vi "Traverse_to_Traverse_Collision.vi"(5 "Current Position  (Tun Coord)":sgl[](array[numeric])=[0.0, 100.0, 40.0], 7 "Traverse Name":string, 10 "Simulate/Run":T1=enum."Run VI", 11 "New Position (Tun Coord)":sgl[](array[numeric])=[0.0, 100.0, 40.0]) -> (1 "Error String":string)   [LabVIEW 2022 SP3]
uses:
  Controls/User_Specific_mode.ctl
  Route mapping/Exclude_cluster.ctl
  Route mapping/Box_size.ctl
  Route mapping/Exclusion_type.ctl
  Globals/Preference_global.vi
panel:
  in  "Max  (Xtunnel - Xtrav1) mm":dbl=2500.0
  out "Z Difference":sgl format="%#.0f"
  out "Xtrav1 - Xtunnel":sgl format="%#.0f"
  out "Static Trav Position (Tun)":sgl[](array[numeric]) format="%#.0f"
  in  "Z Difference":dbl=500.0
  in  "Max  (Xtrav1 - Xtunnel) mm":dbl=30.0
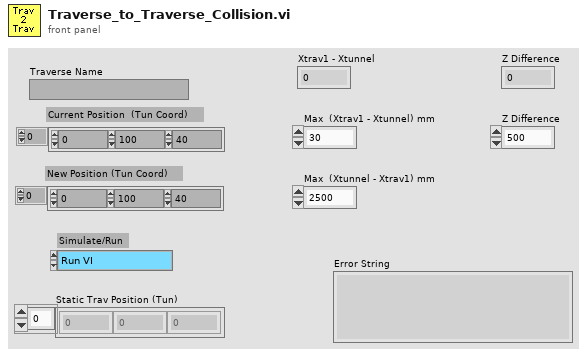
[diagram p1: front panel]
types:
  T1 = typedef "User_Specific_mode.ctl" = enum16{"Check VI only", "Run VI"}
  T2 = typedef "Exclude_cluster.ctl" = cluster{"Sizes":T3, "Name":string, "Exclude Type":T4}
  T3 = typedef "Box_size.ctl" = cluster{"Max":sgl, "Min":sgl}[]
  T4 = typedef "Exclusion_type.ctl" = enum16{"Exclude completely", "Allow only vertical moves"}
  T5 = enum16{"Load setup from excel file", "Save setup to excel file"}
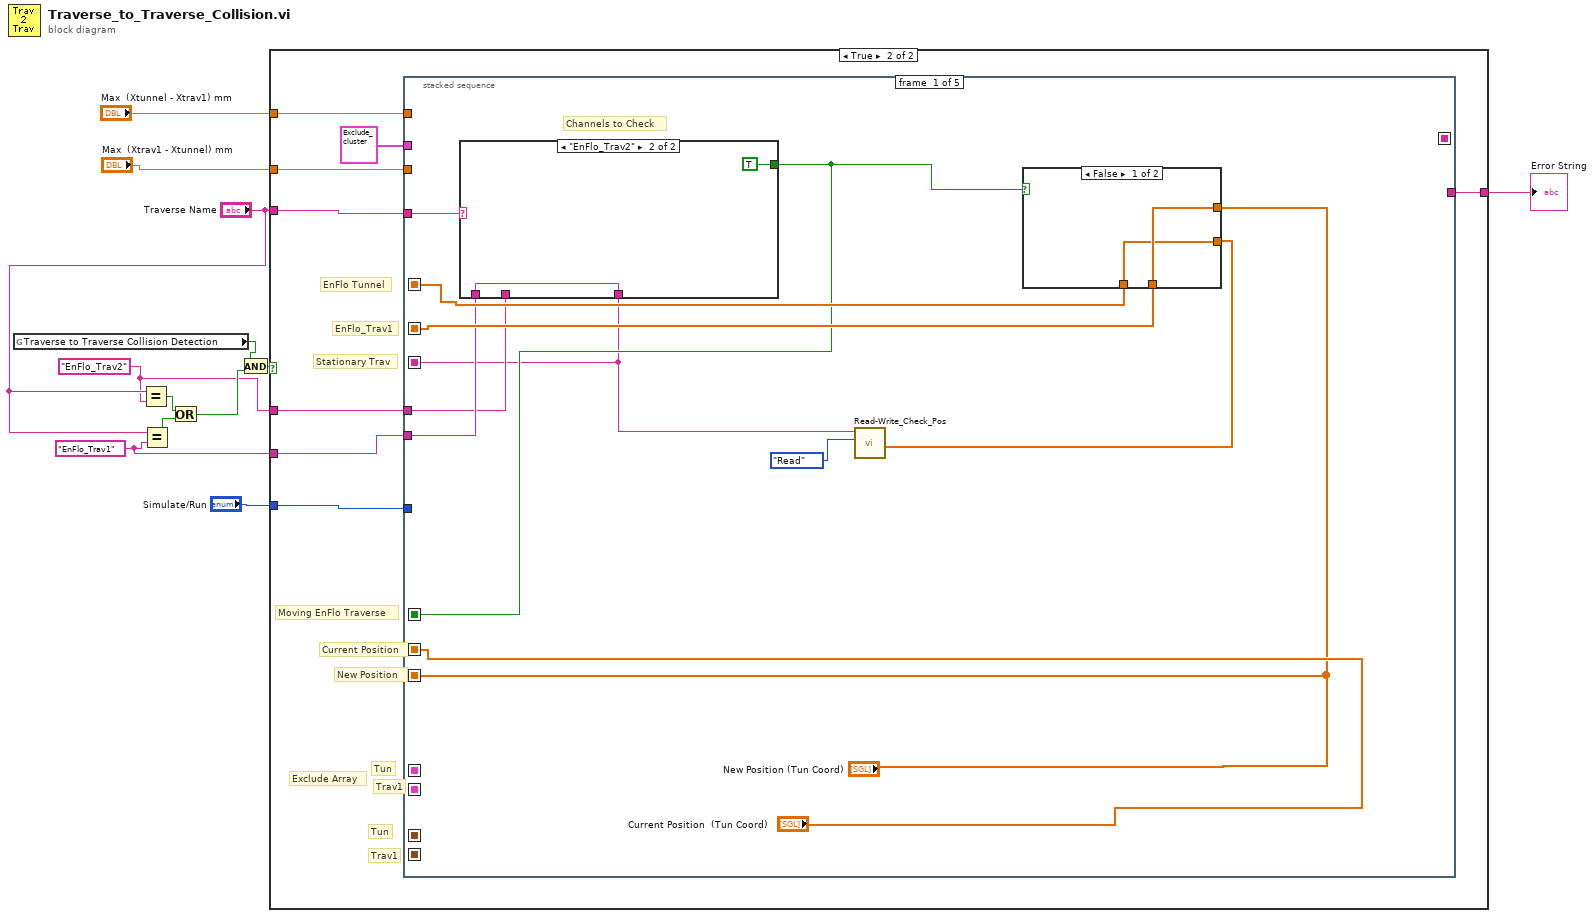
[diagram p0: block diagram]
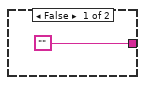
[diagram p2: hidden frame]
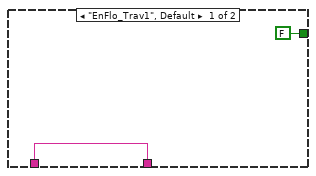
[diagram p4: hidden frame]
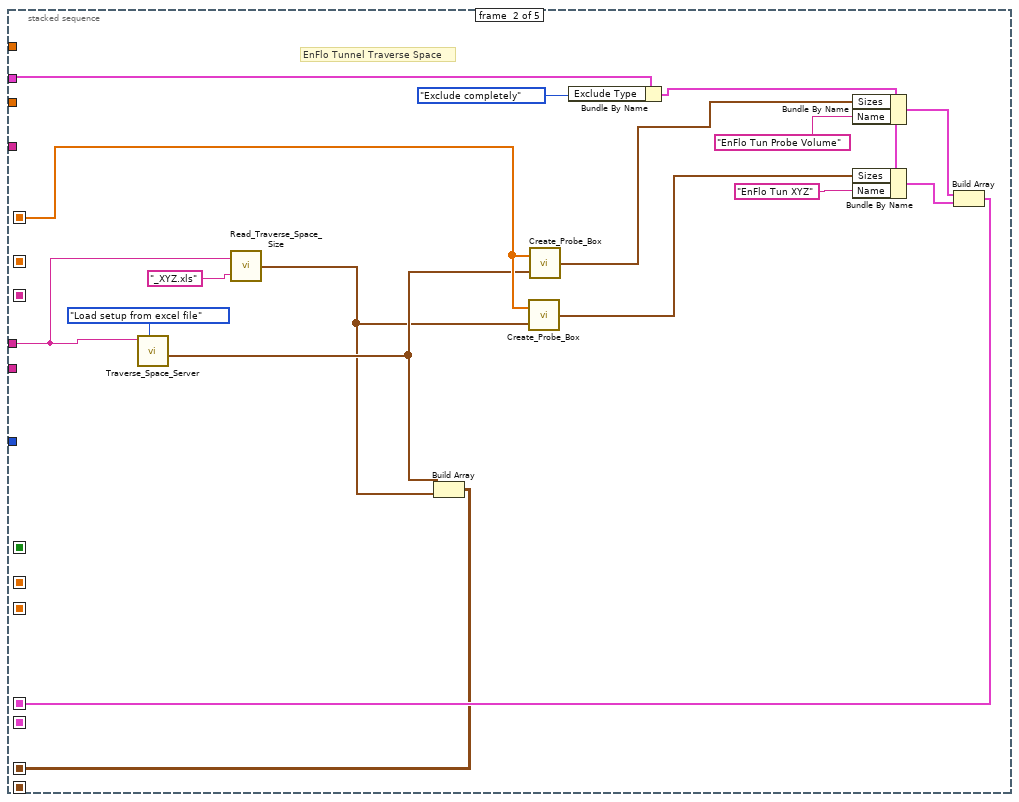
[diagram p5: hidden frame]
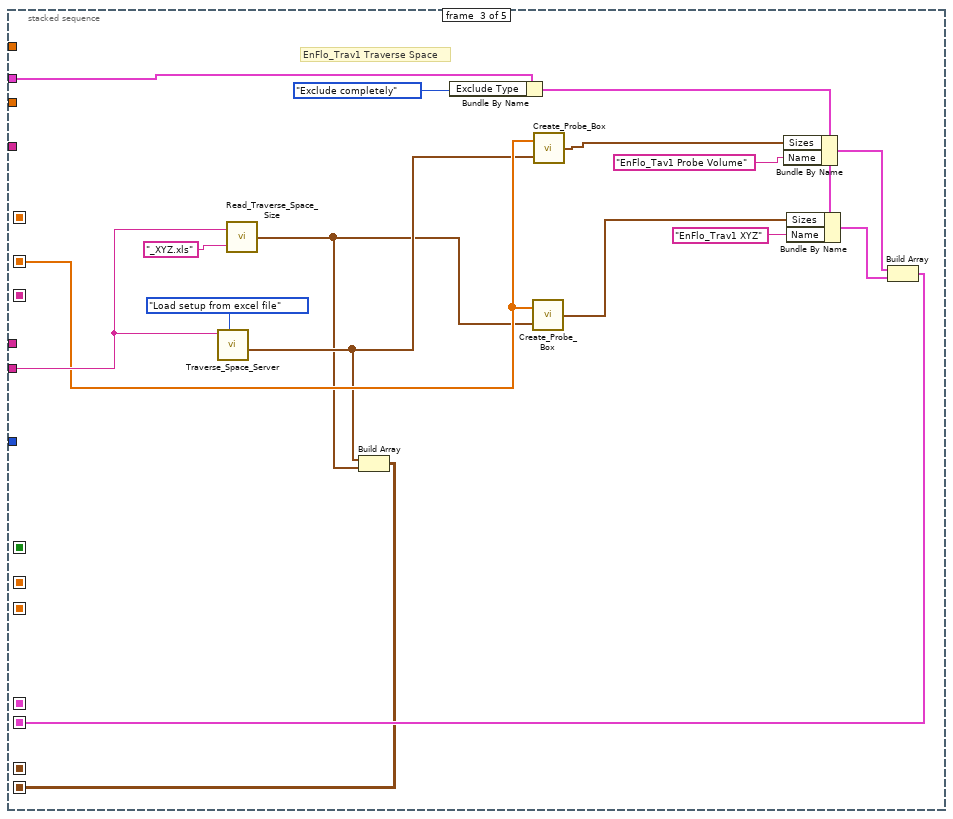
[diagram p6: hidden frame]
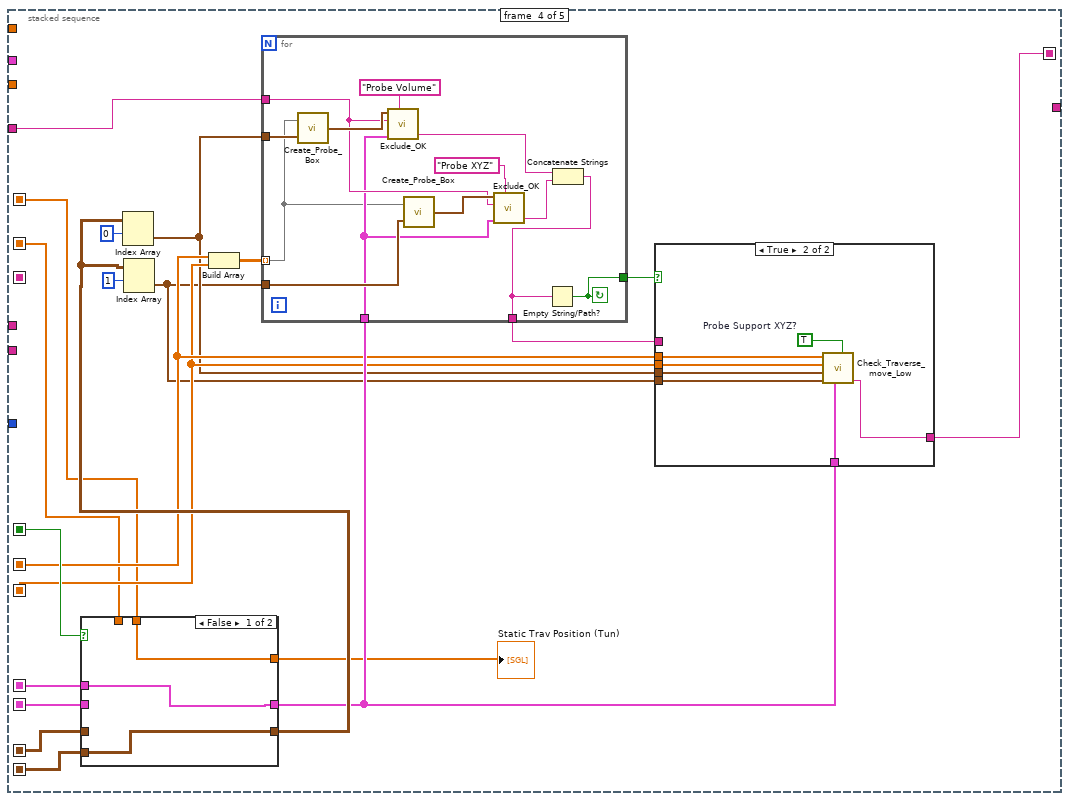
[diagram p7: hidden frame]
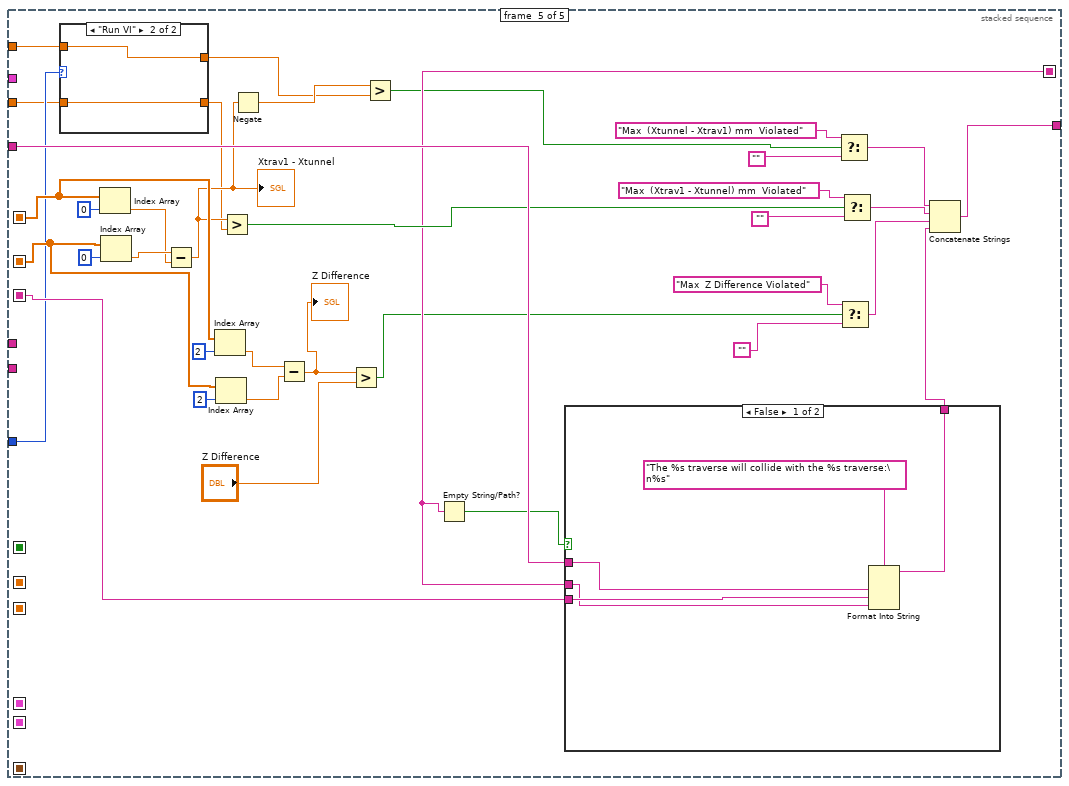
[diagram p10: hidden frame]
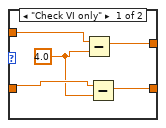
[diagram p11: hidden frame]
diagram:
  w4 = "EnFlo_Trav1" ("Rig Setup")
  w3 = "EnFlo_Trav2" ("Rig Setup")
  n1 = global read "Preference_global.vi" "Traverse to Traverse Collision Detection"() -> (w9:bool)
  n2 = Equal?(x="Traverse Name", y=w3) -> (x = y?=w7:bool)
  n3 = Equal?(x="Traverse Name", y=w4) -> (x = y?=w6:bool)
  n4 = Or(x=w7, y=w6) -> (x .or. y?=w5:bool)
  n5 = And(x=w9, y=w5) -> (x .and. y?=w10:bool)
  n6 = case shown="True" w10 {
    tunnel: "Traverse Name" -> [_ w21]
    tunnel: "Simulate/Run" -> [_ w20]
    tunnel: ["" w19] -> w11
    tunnel: w4 -> [_ w17]
    tunnel: w3 -> [_ w16]
    tunnel: "Max  (Xtrav1 - Xtunnel) mm" -> [_ w15]
    tunnel: "Max  (Xtunnel - Xtrav1) mm" -> [_ w14]
    frame False {
    }
    frame True {
      # "Trav1"
      # "Tun"
      # "Trav1"
      # "Tun"
      # "Stationary Trav"
      # "Moving EnFlo Traverse"
      # "Exclude Array"
      # "Current Position"
      # "New Position"
      # "EnFlo_Trav1"
      # "EnFlo Tunnel"
      n7 = stacked-sequence {
        seq-local: [w32 _ _ _ _] -> [_ w54 _ w75 w144]
        seq-local: [w31 _ _ _ _] -> [_ _ w62 w77 w143]
        seq-local: [w23 _ _ _ _] -> [_ _ _ _ w153]
        seq-local: ["New Position (Tun Coord)" _ _ _ _] -> [_ _ _ w85 _]
        seq-local: [_ _ w71 _ _] -> [_ _ _ w95 _]
        seq-local: [_ w56 _ _ _] -> [_ _ _ w94 _]
        seq-local: ["Current Position  (Tun Coord)" _ _ _ _] -> [_ _ _ w86 _]
        seq-local: [w29 _ _ _ _] -> [_ _ _ w93 _]
        seq-local: [_ _ w58 _ _] -> [_ _ _ w78 _]
        seq-local: [_ w41 _ _ _] -> [_ _ _ w92 _]
        seq-local: [_ _ _ w80 _] -> [_ _ _ _ w147]
        tunnel: w21 -> [w24 _ _ w88 w154]
        tunnel: w20 -> [_ _ _ _ w127]
        tunnel: [_ _ _ _ w155] -> w19
        tunnel: T2 {"Sizes"=[{"Max"=15000.0, "Min"=0.0}, {"Max"=1000.0, "Min"=-1000.0}, {"Max"=300.0, "Min"=0.0}], "Name"="Roughness Elements", "Exclude Type"=enum."Allow only vertical moves"} ("Cluster") -> [_ w50 w66 _ _]
        tunnel: w16 -> [w27 w47 _ _ _]
        tunnel: w17 -> [w28 _ w68 _ _]
        tunnel: w15 -> [_ _ _ _ w123]
        tunnel: w14 -> [_ _ _ _ w125]
        frame #0 {
          # "Channels to Check"
          n8 = case shown="\"EnFlo_Trav2\"" w24 {
            tunnel: [FALSE TRUE] -> w29
            tunnel: [w37 w39] -> w23
            tunnel: w28 -> [_ w39]
            tunnel: w27 -> [w37 _]
            frame "EnFlo_Trav1", Default {
            }
            frame "EnFlo_Trav2" {
            }
          }
          n9 = call "Read-Write_Check_Pos.vi"("Mode"=enum16{"Read", "Write"}."Read", "Traverse Name"=w23) -> ("Position Output"=w25:sgl[])  [unwired: 5 in, 2 out]
          n10 = case shown="False" w29 {
            tunnel: [w33 w36] -> w32
            tunnel: "New Position (Tun Coord)" -> [w34 w36]
            tunnel: [w34 w35] -> w31
            tunnel: w25 -> [w33 w35]
            frame False {
            }
            frame True {
            }
          }
        }
        frame #1 {
          # "EnFlo Tunnel Traverse Space"
          n11 = call "Traverse_Space_Server.vi"("Mode"=T5."Load setup from excel file", "Traverse Name"=w47) -> ("Probe Volume Out"=w43:T3)  [unwired: 4 in, 5 out]
          n12 = call "Read_Traverse_Space_Size.vi"("Space_Name"="_XYZ.xls" ("string"), "Traverse Name"=w47) -> ("Limits out"=w42:T3)
          n13 = Build Array(w43, w42) -> (w41:cluster{"Max":sgl, "Min":sgl}[][])
          n14 = call "Create_Probe_Box.vi"("Probe Volume"=w42, "Probe Position"=w54) -> ("Current Probe Volume"=w44:T3)
          n15 = call "Create_Probe_Box.vi"("Probe Volume"=w43, "Probe Position"=w54) -> ("Current Probe Volume"=w45:T3)
          n16 = Bundle By Name(cluster=w50, "Exclude Type"=Exclusion_type."Exclude completely") -> (w48:T2)
          n17 = Bundle By Name(cluster=w48, "Sizes"=w45, "Name"="EnFlo Tun Probe Volume") -> (w51:T2)
          n18 = Bundle By Name(cluster=w48, "Sizes"=w44, "Name"="EnFlo Tun XYZ") -> (w52:T2)
          n19 = Build Array(w51, w52) -> (w56:T2[])
        }
        frame #2 {
          # "EnFlo_Trav1 Traverse Space"
          n20 = call "Traverse_Space_Server.vi"("Mode"=T5."Load setup from excel file", "Traverse Name"=w68) -> ("Probe Volume Out"=w60:T3)  [unwired: 4 in, 5 out]
          n21 = call "Read_Traverse_Space_Size.vi"("Space_Name"="_XYZ.xls" ("string"), "Traverse Name"=w68) -> ("Limits out"=w59:T3)
          n22 = Build Array(w60, w59) -> (w58:cluster{"Max":sgl, "Min":sgl}[][])
          n23 = Bundle By Name(cluster=w66, "Exclude Type"=Exclusion_type."Exclude completely") -> (w65:T2)
          n24 = call "Create_Probe_Box.vi"("Probe Volume"=w59, "Probe Position"=w62) -> ("Current Probe Volume"=w74:T3)
          n25 = call "Create_Probe_Box.vi"("Probe Volume"=w60, "Probe Position"=w62) -> ("Current Probe Volume"=w61:T3)
          n26 = Bundle By Name(cluster=w65, "Sizes"=w61, "Name"="EnFlo_Tav1 Probe Volume") -> (w64:T2)
          n27 = Bundle By Name(cluster=w65, "Sizes"=w74, "Name"="EnFlo_Trav1 XYZ") -> (w72:T2)
          n28 = Build Array(w64, w72) -> (w71:T2[])
        }
        frame #3 {
          n29 = case shown="False" w93 {
            tunnel: [w119 w122] -> w87
            tunnel: w95 -> [_ w122]
            tunnel: w94 -> [w119 _]
            tunnel: [w118 w121] -> w90
            tunnel: w92 -> [_ w121]
            tunnel: w78 -> [w118 _]
            tunnel: [w117 w120] -> w76
            tunnel: w77 -> [_ w120]
            tunnel: w75 -> [w117 _]
            frame False {
            }
            frame True {
            }
          }
          "Static Trav Position (Tun)" <- w76
          n30 = Index Array(array=w90, index (row)=0) -> (element=w83:cluster{"Max":sgl, "Min":sgl}[])  [unwired: 1 in]
          n31 = Index Array(array=w90, index (row)=1) -> (element=w82:cluster{"Max":sgl, "Min":sgl}[])  [unwired: 1 in]
          n32 = Build Array(w86, w85) -> (w84:sgl[][])
          n33 = for {
            tunnel: w83 -> [w116]
            tunnel: w82 -> [w111]
            tunnel: w88 -> [w110]
            tunnel: w87 -> [w109]
            tunnel: w84 -> [w108] mode=indexing
            tunnel: [w105] -> w81
            tunnel: [w104] -> w79
            stop <- w105 continue-if-true
            n34 = call "Create_Probe_Box.vi"("Probe Volume"=w116, "Probe Position"=w108) -> ("Current Probe Volume"=w115:T3)
            n35 = call "Exclude_OK.vi"("Probe Volume"=w115, "Traverse Name"=w110, "Exclude Array"=w109, "Volume Name"="Probe Volume") -> ("Error Comments"=w106:string)  [unwired: 1 in, 2 out]
            n36 = call "Create_Probe_Box.vi"("Probe Volume"=w111, "Probe Position"=w108) -> ("Current Probe Volume"=w112:T3)
            n37 = call "Exclude_OK.vi"("Probe Volume"=w112, "Traverse Name"=w110, "Exclude Array"=w109, "Volume Name"="Probe XYZ") -> ("Error Comments"=w107:string)  [unwired: 1 in, 2 out]
            n38 = Concatenate Strings(w106, w107) -> (w104:string)
            n39 = Empty String/Path?(string/path=w104) -> (empty?=w105:bool)
          }
          n40 = case shown="True" w81 {
            tunnel: w87 -> [_ w102]
            tunnel: w86 -> [_ w101]
            tunnel: w85 -> [_ w100]
            tunnel: w83 -> [_ w99]
            tunnel: w82 -> [_ w98]
            tunnel: [w96 w97] -> w80
            tunnel: w79 -> [w96 _]
            frame False {
            }
            frame True {
              w103 = TRUE  # Probe Support XYZ?
              n41 = call "Check_Traverse_move_Low.vi"("Probe Support XYZ?"=w103, "Exclude Array"=w102, "Probe Support"=w98, "Probe Volume"=w99, "New Position"=w100, "Current position"=w101) -> ("Error Comments"=w97:string)  [unwired: 2 in, 1 out]
            }
          }
        }
        frame #4 {
          n42 = case shown="\"Run VI\"" w127 {
            tunnel: [w163 w166] -> w126
            tunnel: w125 -> [w164 w166]
            tunnel: [w161 w165] -> w124
            tunnel: w123 -> [w162 w165]
            frame "Check VI only" {
              w160 = 4.0 ("y")
              n43 = Subtract(x=w164, y=w160) -> (x-y=w163:dbl)
              n44 = Subtract(x=w162, y=w160) -> (x-y=w161:dbl)
            }
            frame "Run VI" {
            }
          }
          n45 = Index Array(array=w144, index=0) -> (element=w156:sgl)
          n46 = Index Array(array=w143, index=0) -> (element=w157:sgl)
          n47 = Subtract(x=w157, y=w156) -> (x-y=w133:sgl)
          "Xtrav1 - Xtunnel" <- w133
          n48 = Index Array(array=w144, index=2) -> (element=w142:sgl)
          n49 = Index Array(array=w143, index=2) -> (element=w141:sgl)
          n50 = Greater?(x=w133, y=w124) -> (0:w150:bool)
          n51 = Negate(x=w133) -> (-x=w132:sgl)
          n52 = Subtract(x=w142, y=w141) -> (x-y=w134:sgl)
          "Z Difference" <- w134
          n53 = Greater?(x=w134, y="Z Difference") -> (0:w135:bool)
          n54 = Greater?(x=w132, y=w126) -> (0:w128:bool)
          n55 = Empty String/Path?(string/path=w147) -> (empty?=w148:bool)
          n56 = case shown="False" w148 {
            tunnel: [w169 w172] -> w137
            tunnel: w147 -> [w167 w172]
            tunnel: w154 -> [w168 _]
            tunnel: w153 -> [w170 _]
            frame False {
              n57 = Format Into String(format string="The %s traverse will collide with the %s traverse:\n%s" ("Format String"), w168, w170, w167) -> (resulting string=w169:string)  [unwired: 2 in, 1 out]
            }
            frame True {
            }
          }
          n58 = Select(t="Max  (Xtunnel - Xtrav1) mm  Violated", s=w128, f="") -> (s? t:f=w129:string)
          n59 = Select(t="Max  Z Difference Violated", s=w135, f="") -> (s? t:f=w136:string)
          n60 = Select(t="Max  (Xtrav1 - Xtunnel) mm  Violated", s=w150, f="") -> (s? t:f=w149:string)
          n61 = Concatenate Strings(w129, w149, w136, w137) -> (w155:string)
        }
      }
    }
  }
  "Error String" <- w11
